vi "Read Task Manager Error.vi"(8 "error in (no error)":errorcluster, 11 "Error Task Manager in":refnum<class "Error Task Manager.lvclass">) -> (0 "error out":errorcluster, 2 "Task Manager Error":refnum<user-event>, 3 "Error Task Manager out":refnum<class "Error Task Manager.lvclass">)   [LabVIEW 2013, in "Error Task Manager.lvlib" / "Error Task Manager.lvclass"]
uses:
  Error Task Manager.lvclass
  Error Task Manager.lvclass/Error Task Manager.ctl
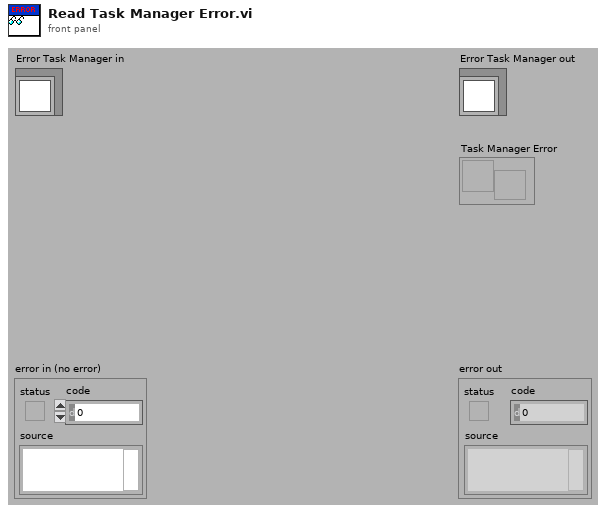
[diagram p1: front panel]
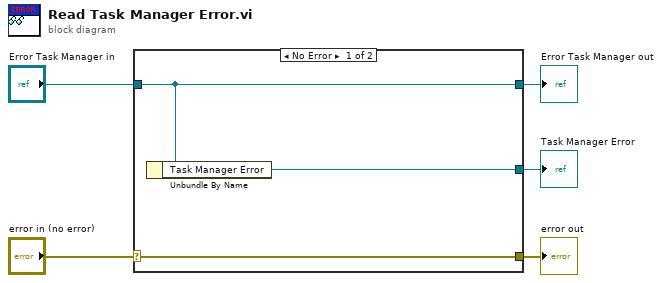
[diagram p0: block diagram]
diagram:
  n1 = case shown="No Error" "error in (no error)" {
    selector: "error in (no error)" -> [w8 w9]
    tunnel: [w8 w9] -> w4
    tunnel: [w7 w10] -> w2
    tunnel: "Error Task Manager in" -> [w7 w10]
    tunnel: [w6 _] -> w1
    frame No Error {
      n2 = Unbundle By Name(w7) -> ("Task Manager Error"=w6:refnum<user-event>)
    }
    frame Error {
    }
  }
  "error out" <- w4
  "Error Task Manager out" <- w2
  "Task Manager Error" <- w1
